vi "ConsumeWsp.vi"(8 "error in (no error)":errorcluster, 11 "PathTokenizer in":refnum<class "PathTokenizer.lvclass">) -> (0 "error out":errorcluster, 3 "PathTokenizer out":refnum<class "PathTokenizer.lvclass">)   [LabVIEW 2019, in "PathTokenizer.lvclass"]
uses:
  PathTokenizer.lvclass
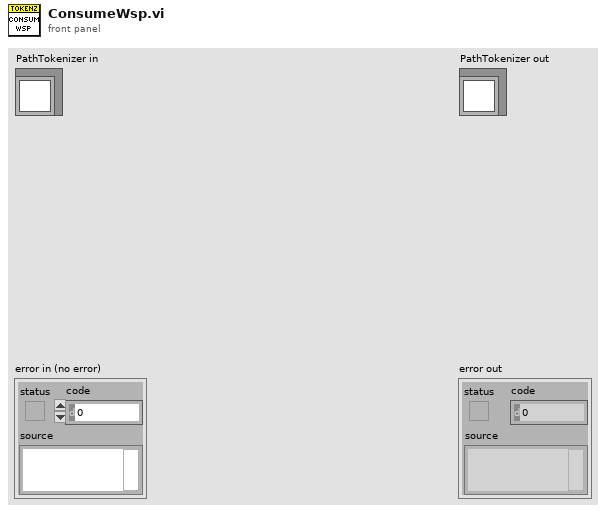
[diagram p1: front panel]
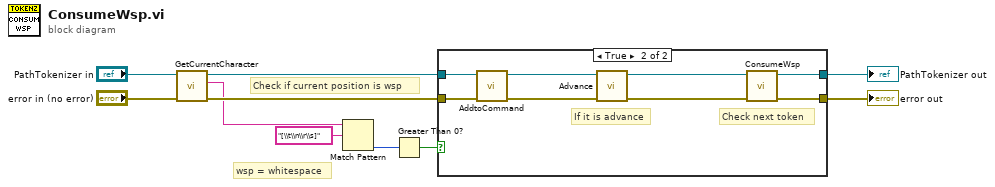
[diagram p0: block diagram]
diagram:
  # "wsp = whitespace"
  # "Check if current position is wsp"
  n1 = call "GetCurrentCharacter.vi"("error in (no error)"="error in (no error)", "PathTokenizer in"="PathTokenizer in") -> ("error out"=w4:errorcluster, "Current Character"=w2:string, "PathTokenizer out"=w5:refnum<class "PathTokenizer.lvclass">)  [unwired: 7 in]
  n2 = Match Pattern(string=w2, regular expression="[\\t\\n\\r\\s]") -> (offset past match=w8:i32)  [unwired: 1 in, 3 out]
  n3 = Greater Than 0?(x=w8) -> (x > 0?=w7:bool)
  n4 = case shown="True" w7 {
    tunnel: w5 -> [w12 w15]
    tunnel: [w12 w20] -> w10
    tunnel: w4 -> [w11 w14]
    tunnel: [w11 w19] -> w6
    frame False {
      # "If not, nothing to consume"
    }
    frame True {
      # "If it is advance"
      # "Check next token"
      n5 = call "AddtoCommand.vi"("error in (no error)"=w14, "PathTokenizer in"=w15) -> ("error out"=w13:errorcluster, "PathTokenizer out"=w16:refnum<class "PathTokenizer.lvclass">)  [unwired: 8 in]
      n6 = call "Advance.vi"("error in (no error)"=w13, "PathTokenizer in"=w16) -> ("error out"=w17:errorcluster, "PathTokenizer out"=w18:refnum<class "PathTokenizer.lvclass">)  [unwired: 8 in]
      n7 = call "ConsumeWsp.vi"("error in (no error)"=w17, "PathTokenizer in"=w18) -> ("error out"=w19:errorcluster, "PathTokenizer out"=w20:refnum<class "PathTokenizer.lvclass">)  [unwired: 8 in]
    }
  }
  "error out" <- w6
  "PathTokenizer out" <- w10
